vi "DestroyListenerProcess.vi"(8 "error in (no error)":errorcluster, 10 "process name":string, 11 "Qbus in":refnum<class "Qbus.lvclass">) -> (0 "error in (no error)":errorcluster, 3 "Qbus out":refnum<class "Qbus.lvclass">)   [LabVIEW 2017, in "Qbus.lvclass"]
doc: "Closes the message queue and other resources that integrate a process with Qbus."
uses:
  <vilib>/addons/Qbus/Qbus.lvclass
  <vilib>/addons/Qbus/Qbus.lvclass/Qbus.ctl
  <vilib>/addons/Qbus/controls/message.ctl
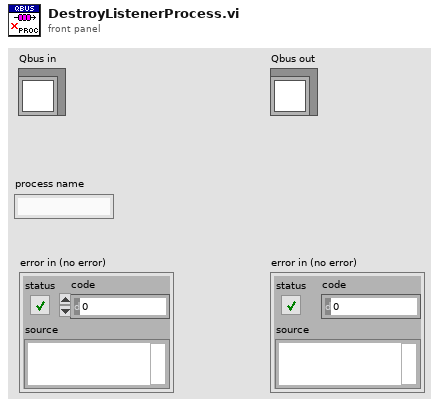
[diagram p1: front panel]
types:
  T1 = typedef "Qbus.lvclass/data.ctl" = cluster{"Queues":variant, "Subscriptions":variant, "MasterQ":string}
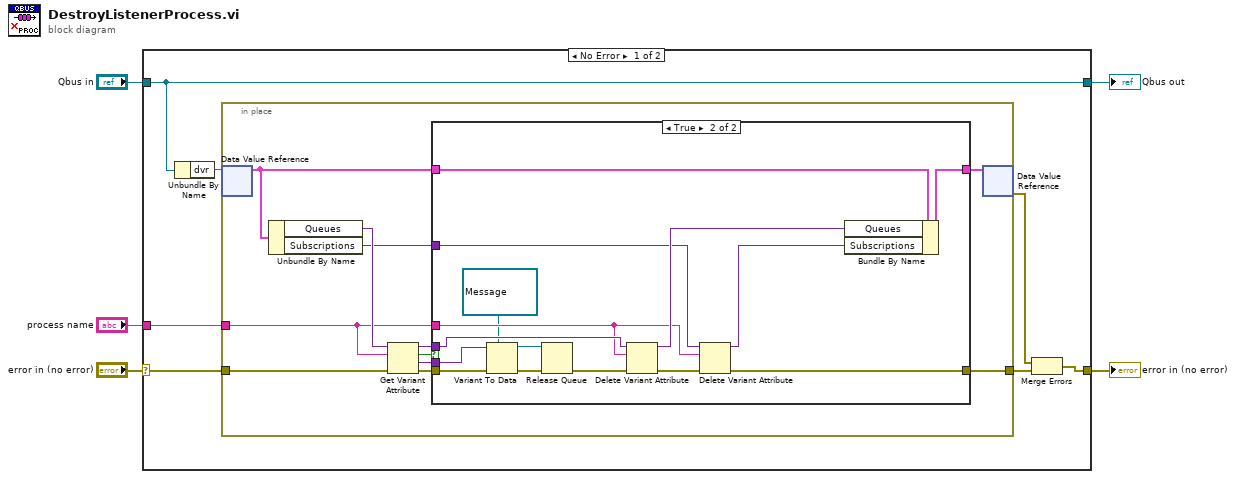
[diagram p0: block diagram]
diagram:
  n1 = case shown="No Error" "error in (no error)" {
    selector: "error in (no error)" -> [w8 w42]
    tunnel: [w7 w42] -> w4
    tunnel: [w12 w41] -> w2
    tunnel: "Qbus in" -> [w12 w41]
    tunnel: "process name" -> [w10 _]
    frame No Error {
      n2 = Unbundle By Name(w12) -> ("dvr"=w11:refnum<data-value>)
      n3 = in-place {
        in-place-border: w8 -> [w23]
        in-place-border: w10 -> [w15]
        in-place-border: [w14] -> w6
        n4 = in-place-dvr #1(w11) -> (w19:T1)  [unwired: 1 out]
        n5 = Unbundle By Name(w19) -> ("Queues"=w18:variant, "Subscriptions"=w16:variant)
        n6 = Get Variant Attribute(Variant=w18, name=w15, error in=w23) -> (duplicate Variant=w17:variant, found=w22:bool, value=w13:variant, error out=w21:errorcluster)  [unwired: 1 in]
        n7 = case shown="True" w22 {
          tunnel: w21 -> [w24 w31]
          tunnel: [w25 w39] -> w20
          tunnel: w19 -> [w25 w40]
          tunnel: w17 -> [_ w37]
          tunnel: w16 -> [_ w35]
          tunnel: w15 -> [_ w33]
          tunnel: [w24 w26] -> w14
          tunnel: w13 -> [_ w30]
          frame False {
          }
          frame True {
            n8 = Variant To Data(error in=w31, type=refnum<queue> refnum ("queue out"), Variant=w30) -> (data=w27:refnum<queue>, error out=w29:errorcluster)
            n9 = Release Queue(queue=w27, error in (no error)=w29) -> (error out=w28:errorcluster)  [unwired: 1 in, 2 out]
            n10 = Delete Variant Attribute(4:w28, 6:w33, 7:w37) -> (0:w38:errorcluster, 3:w36:variant)  [unwired: 1 out]
            n11 = Delete Variant Attribute(4:w38, 6:w33, 7:w35) -> (0:w26:errorcluster, 3:w34:variant)  [unwired: 1 out]
            n12 = Bundle By Name(cluster=w40, "Queues"=w36, "Subscriptions"=w34) -> (w39:T1)
          }
        }
        n13 = in-place-dvr #1(w20) -> (w9:errorcluster)  [unwired: 1 out]
      }
      n14 = Merge Errors(w9, w6) -> (w7:errorcluster)
    }
    frame Error {
    }
  }
  "error in (no error)" <- w4
  "Qbus out" <- w2
